vi "poly_control_value_from_name_caller_single.vi"(8 "error in (no error)":errorcluster, 9 "control name":string, 10 "name of caller in (your caller)":string) -> (0 "error out":errorcluster, 1 "Value":variant, 4 "found?":bool, 5 "ctrl ref":refnum<vi>)   [LabVIEW 2015]
uses:
  poly_ref_tools_eco_plus.vi
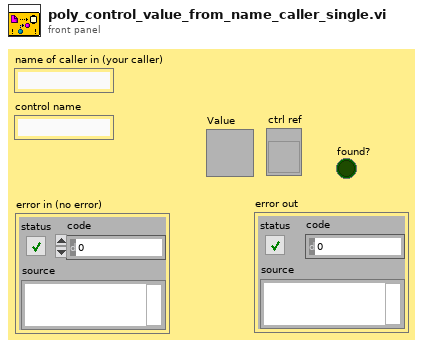
[diagram p1: front panel]
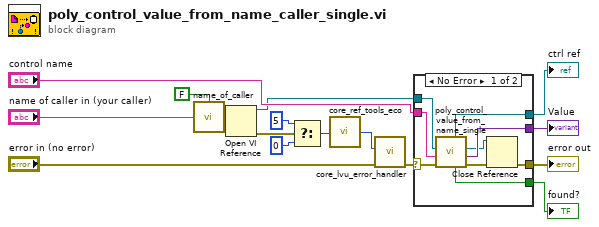
[diagram p0: block diagram]
diagram:
  n1 = call "name_of_caller.vi"("is in inlined vi? (F)"=FALSE, "name of caller in"="name of caller in (your caller)") -> ("name of caller out"=w11:string)  [unwired: 2 in]
  n2 = Open VI Reference(vi path=w11) -> (vi reference=w10:refnum<vi>, error out=w7:errorcluster)  [unwired: 5 in]
  n3 = Select(t=5, s=w7, f=0) -> (s? t:f=w2:i32)
  n4 = call-poly "core_ref_tools_eco.vi"("code (w/out eco)"=w2) -> ("code (+ eco)"=w1:i32)  [unwired: 4 in]
  n5 = call "core_lvu_error_handler.vi"("error in (no error)"="error in (no error)", "code (0 = no error)"=w1) -> ("error out"=w3:errorcluster)  [unwired: 8 in, 1 out]
  n6 = case shown="No Error" w3 {
    selector: w3 -> [w17 w26]
    tunnel: [w25 _] -> w16
    tunnel: [w24 _] -> w15
    tunnel: [w23 _] -> w14
    tunnel: "control name" -> [w22 _]
    tunnel: w10 -> [w21 _]
    tunnel: [w19 w26] -> w9
    frame No Error {
      n7 = call "poly_control_value_from_name_single.vi"("error in (no error)"=w17, "control name"=w22, "vi ref"=w21) -> ("error out"=w20:errorcluster, "Value"=w25:variant, "vi ref dup"=w18:refnum<vi>, "found?"=w23:bool, "ctrl ref"=w24:refnum<vi>)  [unwired: 4 in]
      n8 = Close Reference(reference=w18, error in (no error)=w20) -> (error out=w19:errorcluster)
    }
    frame Error {
    }
  }
  "ctrl ref" <- w15
  "error out" <- w9
  "found?" <- w14
  "Value" <- w16
